vi "Message Box.vi"(2 "path":path, 3 "Text In":string) -> (0 "stop 2":bool, 1 "Text Out":string)   [LabVIEW 2012]
panel:
  in  "stop":bool
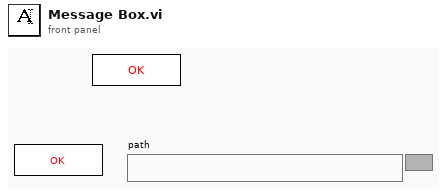
[diagram p1: front panel]
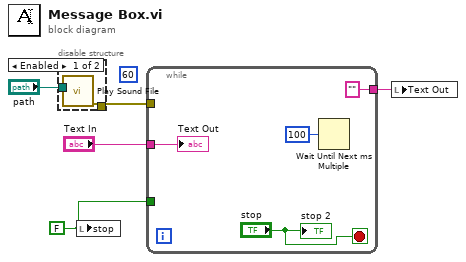
[diagram p0: block diagram]
diagram:
  (unwired) 60
  w5 = FALSE ("stop")
  n1 = disable-structure shown="Enabled" {
    disable-tunnel: [w7 _] -> w4
    disable-tunnel: "path" -> [w6 _]
    frame Enabled {
      n2 = call <vilib>:"Play Sound File.vi"("path"=w6) -> ("error out"=w7:errorcluster)  [unwired: 9 in, 1 out]
    }
    frame Disabled {
    }
  }
  n3 = local write "stop"(w5) -> ()
  n4 = while {
    tunnel: w5 -> [_]
    tunnel: w4 -> [_]
    tunnel: "Text In" -> [w10]
    tunnel: ["" ("Text Out")] -> w1
    stop <- "stop" stop-if-true
    n5 = Wait Until Next ms Multiple(millisecond multiple=u32 100) -> ()  [unwired: 1 out]
    "Text Out" <- w10
    "stop 2" <- "stop"
  }
  n6 = local write "Text Out"(w1) -> ()
